vi "rtlsdr_config.vi"(0 "ref in":refnum<k5>, 1 "LO frequency":i32=-2147483647, 2 "Samplerate":i32=-2147483647, 3 "Autogain":i32=-2147483647, 4 "Gain":i32=-2147483647, 5 "error in":errorcluster, 6 "IF stage gain":i32=-2147483647, 7 "PPM":i32=-2147483647, 8 "Test mode":i32=-2147483647, 9 "RTL XTAL frequency":i32=-2147483647, 10 "AGC mode":i32=-2147483647, 11 "Tuner XTAL frequency":i32=-2147483647, 12 "Direct sampling":i32=-2147483647, 13 "Tuner gain by index":i32=-2147483647, 18 "Offset tuning":i32=-2147483647) -> (14 "ref out":refnum<k5>, 19 "error out":errorcluster)   [LabVIEW 2011]
panel:
  # "Inputs:"
  # "Outputs:"
  # "This routine will set parameters on an RTLSDR device. It won't set those parameters that don't have their input terminals wired."
  # "For boolean parameters, write integer 1 or 0 to the input terminal. (There's a built-in function to do that conversion from boolean.)"
  # "For more information about all the parameters, dig in the rtl_tcp.c source:"
  # "http://cgit.osmocom.org/rtl-sdr/tree/src/rtl_tcp.c"
  # "Search for \"cmd.cmd\" to find the place where these are processed. For most of the time, you might use only a few of these commands."
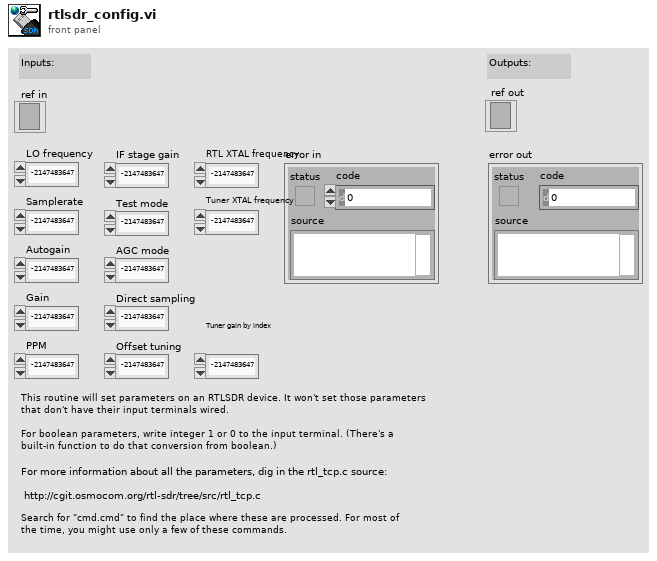
[diagram p1: front panel]
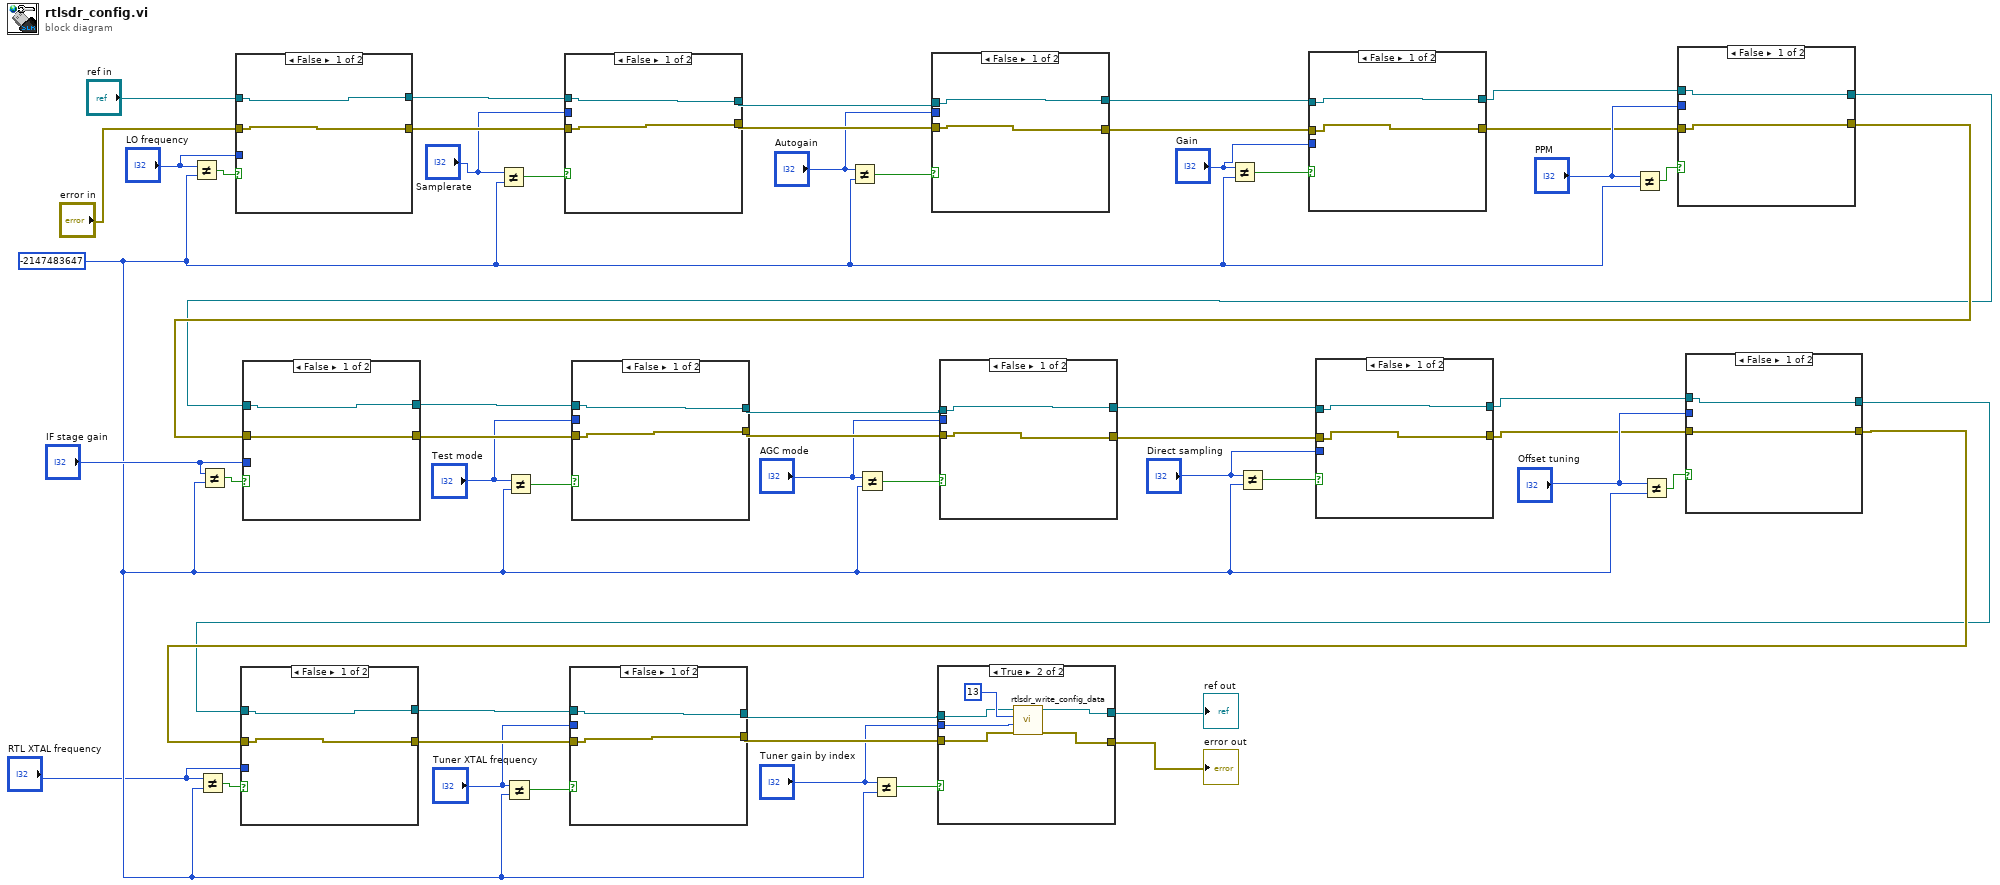
[diagram p0: block diagram]
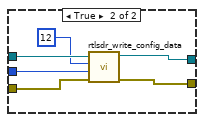
[diagram p3: hidden frame]
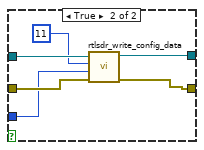
[diagram p4: hidden frame]
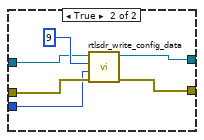
[diagram p5: hidden frame]
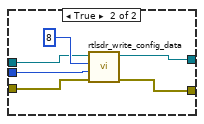
[diagram p6: hidden frame]
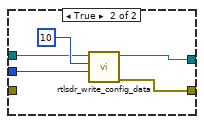
[diagram p7: hidden frame]
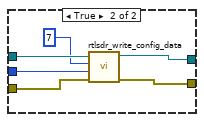
[diagram p8: hidden frame]
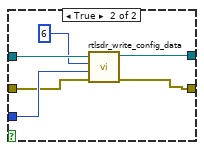
[diagram p9: hidden frame]
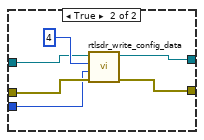
[diagram p10: hidden frame]
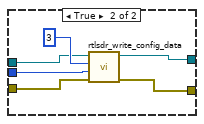
[diagram p11: hidden frame]
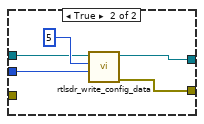
[diagram p12: hidden frame]
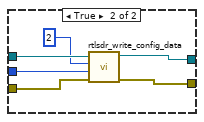
[diagram p13: hidden frame]
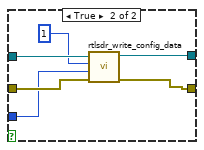
[diagram p14: hidden frame]
diagram:
  w8 = -2147483647 ("y")
  n1 = Not Equal?(x="LO frequency", y=w8) -> (x != y?=w55:bool)
  n2 = Not Equal?(x="RTL XTAL frequency", y=w8) -> (x != y?=w18:bool)
  n3 = Not Equal?(x="IF stage gain", y=w8) -> (x != y?=w36:bool)
  n4 = case shown="False" w55 {
    tunnel: "ref in" -> [w56 w63]
    tunnel: "error in" -> [w57 w62]
    tunnel: "LO frequency" -> [_ w59]
    tunnel: [w56 w61] -> w50
    tunnel: [w57 w60] -> w51
    frame False {
    }
    frame True {
      n5 = call "rtlsdr_write_config_data.vi"("error in (no error)"=w62, "input data"=w59, "parameter select"=u8 1, "ref in"=w63) -> ("error out"=w60:errorcluster, "ref out"=w61:refnum<k5>)  [unwired: 6 in]
    }
  }
  n6 = Not Equal?(x="Samplerate", y=w8) -> (x != y?=w49:bool)
  n7 = Not Equal?(x="Tuner XTAL frequency", y=w8) -> (x != y?=w15:bool)
  n8 = Not Equal?(x="Test mode", y=w8) -> (x != y?=w33:bool)
  n9 = case shown="False" w49 {
    tunnel: w50 -> [w64 w71]
    tunnel: w51 -> [w65 w70]
    tunnel: [w64 w69] -> w45
    tunnel: [w65 w66] -> w44
    tunnel: "Samplerate" -> [_ w67]
    frame False {
    }
    frame True {
      n10 = call "rtlsdr_write_config_data.vi"("error in (no error)"=w70, "input data"=w67, "parameter select"=u8 2, "ref in"=w71) -> ("error out"=w66:errorcluster, "ref out"=w69:refnum<k5>)  [unwired: 6 in]
    }
  }
  n11 = Not Equal?(x="Autogain", y=w8) -> (x != y?=w43:bool)
  n12 = Not Equal?(x="AGC mode", y=w8) -> (x != y?=w29:bool)
  n13 = Not Equal?(x="Tuner gain by index", y=w8) -> (x != y?=w12:bool)
  n14 = case shown="False" w43 {
    tunnel: w45 -> [w72 w75]
    tunnel: w44 -> [w73 w79]
    tunnel: [w72 w78] -> w41
    tunnel: [w73 w76] -> w39
    tunnel: "Autogain" -> [_ w74]
    frame False {
    }
    frame True {
      n15 = call "rtlsdr_write_config_data.vi"("error in (no error)"=w79, "input data"=w74, "parameter select"=u8 3, "ref in"=w75) -> ("error out"=w76:errorcluster, "ref out"=w78:refnum<k5>)  [unwired: 6 in]
    }
  }
  n16 = Not Equal?(x="Gain", y=w8) -> (x != y?=w38:bool)
  n17 = Not Equal?(x="Direct sampling", y=w8) -> (x != y?=w25:bool)
  n18 = case shown="False" w38 {
    tunnel: w41 -> [w80 w83]
    tunnel: w39 -> [w81 w87]
    tunnel: [w80 w86] -> w40
    tunnel: [w81 w84] -> w2
    tunnel: "Gain" -> [_ w82]
    frame False {
    }
    frame True {
      n19 = call "rtlsdr_write_config_data.vi"("error in (no error)"=w87, "input data"=w82, "parameter select"=u8 4, "ref in"=w83) -> ("error out"=w84:errorcluster, "ref out"=w86:refnum<k5>)  [unwired: 6 in]
    }
  }
  n20 = Not Equal?(x="PPM", y=w8) -> (x != y?=w47:bool)
  n21 = Not Equal?(x="Offset tuning", y=w8) -> (x != y?=w32:bool)
  n22 = case shown="False" w47 {
    tunnel: [w88 w94] -> w11
    tunnel: [w89 w92] -> w24
    tunnel: "PPM" -> [_ w91]
    tunnel: w40 -> [w88 w90]
    tunnel: w2 -> [w89 _]
    frame False {
    }
    frame True {
      n23 = call "rtlsdr_write_config_data.vi"("input data"=w91, "parameter select"=u8 5, "ref in"=w90) -> ("error out"=w92:errorcluster, "ref out"=w94:refnum<k5>)  [unwired: 7 in]
    }
  }
  n24 = case shown="False" w36 {
    tunnel: w11 -> [w96 w102]
    tunnel: "IF stage gain" -> [_ w99]
    tunnel: [w96 w101] -> w34
    tunnel: [w95 w100] -> w35
    tunnel: w24 -> [w95 w97]
    frame False {
    }
    frame True {
      n25 = call "rtlsdr_write_config_data.vi"("error in (no error)"=w97, "input data"=w99, "parameter select"=u8 6, "ref in"=w102) -> ("error out"=w100:errorcluster, "ref out"=w101:refnum<k5>)  [unwired: 6 in]
    }
  }
  n26 = case shown="False" w33 {
    tunnel: w34 -> [w103 w110]
    tunnel: w35 -> [w104 w109]
    tunnel: [w103 w108] -> w31
    tunnel: [w104 w105] -> w30
    tunnel: "Test mode" -> [_ w106]
    frame False {
    }
    frame True {
      n27 = call "rtlsdr_write_config_data.vi"("error in (no error)"=w109, "input data"=w106, "parameter select"=u8 7, "ref in"=w110) -> ("error out"=w105:errorcluster, "ref out"=w108:refnum<k5>)  [unwired: 6 in]
    }
  }
  n28 = case shown="False" w29 {
    tunnel: w31 -> [w111 w114]
    tunnel: w30 -> [w112 w118]
    tunnel: [w111 w117] -> w28
    tunnel: [w112 w115] -> w26
    tunnel: "AGC mode" -> [_ w113]
    frame False {
    }
    frame True {
      n29 = call "rtlsdr_write_config_data.vi"("error in (no error)"=w118, "input data"=w113, "parameter select"=u8 8, "ref in"=w114) -> ("error out"=w115:errorcluster, "ref out"=w117:refnum<k5>)  [unwired: 6 in]
    }
  }
  n30 = case shown="False" w25 {
    tunnel: w28 -> [w119 w122]
    tunnel: w26 -> [w120 w126]
    tunnel: [w119 w125] -> w27
    tunnel: [w120 w123] -> w1
    tunnel: "Direct sampling" -> [_ w121]
    frame False {
    }
    frame True {
      n31 = call "rtlsdr_write_config_data.vi"("error in (no error)"=w126, "input data"=w121, "parameter select"=u8 9, "ref in"=w122) -> ("error out"=w123:errorcluster, "ref out"=w125:refnum<k5>)  [unwired: 6 in]
    }
  }
  n32 = case shown="False" w32 {
    tunnel: [w127 w133] -> w9
    tunnel: [w128 w131] -> w10
    tunnel: "Offset tuning" -> [_ w130]
    tunnel: w27 -> [w127 w129]
    tunnel: w1 -> [w128 _]
    frame False {
    }
    frame True {
      n33 = call "rtlsdr_write_config_data.vi"("input data"=w130, "parameter select"=u8 10, "ref in"=w129) -> ("error out"=w131:errorcluster, "ref out"=w133:refnum<k5>)  [unwired: 7 in]
    }
  }
  n34 = case shown="False" w18 {
    tunnel: w9 -> [w134 w141]
    tunnel: w10 -> [w135 w140]
    tunnel: "RTL XTAL frequency" -> [_ w137]
    tunnel: [w134 w139] -> w16
    tunnel: [w135 w138] -> w17
    frame False {
    }
    frame True {
      n35 = call "rtlsdr_write_config_data.vi"("error in (no error)"=w140, "input data"=w137, "parameter select"=u8 11, "ref in"=w141) -> ("error out"=w138:errorcluster, "ref out"=w139:refnum<k5>)  [unwired: 6 in]
    }
  }
  n36 = case shown="False" w15 {
    tunnel: w16 -> [w142 w149]
    tunnel: w17 -> [w143 w148]
    tunnel: [w142 w147] -> w14
    tunnel: [w143 w144] -> w13
    tunnel: "Tuner XTAL frequency" -> [_ w145]
    frame False {
    }
    frame True {
      n37 = call "rtlsdr_write_config_data.vi"("error in (no error)"=w148, "input data"=w145, "parameter select"=u8 12, "ref in"=w149) -> ("error out"=w144:errorcluster, "ref out"=w147:refnum<k5>)  [unwired: 6 in]
    }
  }
  n38 = case shown="True" w12 {
    tunnel: w14 -> [w150 w153]
    tunnel: w13 -> [w151 w157]
    tunnel: [w150 w156] -> w3
    tunnel: [w151 w154] -> w4
    tunnel: "Tuner gain by index" -> [_ w152]
    frame False {
    }
    frame True {
      n39 = call "rtlsdr_write_config_data.vi"("error in (no error)"=w157, "input data"=w152, "parameter select"=u8 13, "ref in"=w153) -> ("error out"=w154:errorcluster, "ref out"=w156:refnum<k5>)  [unwired: 6 in]
    }
  }
  "ref out" <- w3
  "error out" <- w4
